vi "M9290A Measure Peak.vi"(7 "Route Names":string[](array[string]), 8 "error in":errorcluster, 10 "Center Frequency (100 MHz)":dbl=1000000000.0, 11 "VISA resource name":refnum<visa-resource-name>="ZVL") -> (0 "error out":errorcluster, 2 "Marker Amplitude (Cal)":dbl, 3 "Marker Amplitude (Raw)":dbl)   [LabVIEW 2015]
uses:
  <instrlib>/Agilent MXA Series/Public/Data/Read Trace (Swept SA).vi
panel:
  out "VISA resource name out":refnum<visa-resource-name>
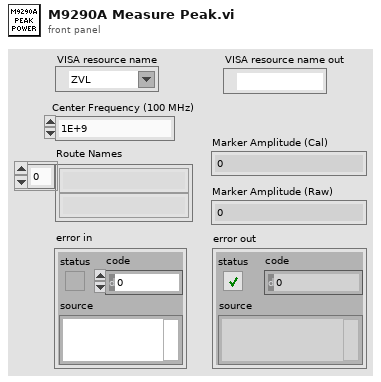
[diagram p1: front panel]
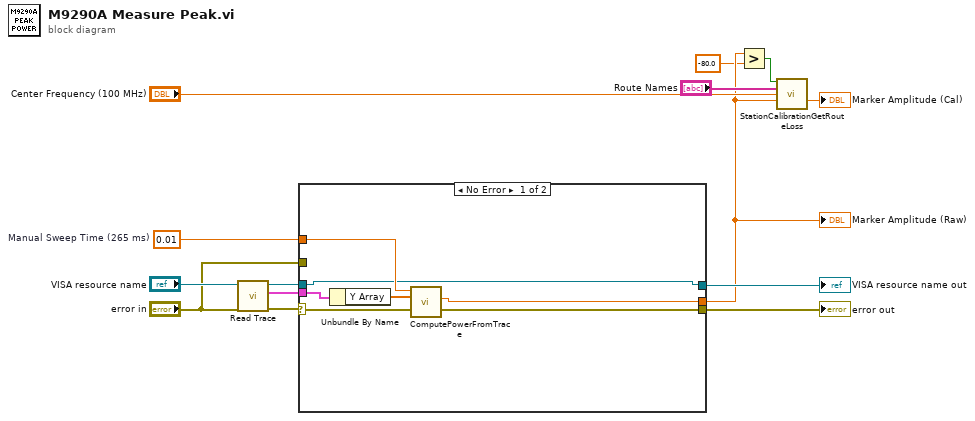
[diagram p0: block diagram]
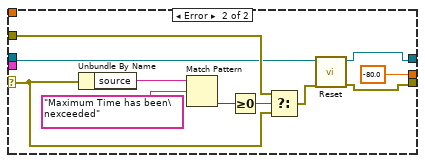
[diagram p2: hidden frame]
diagram:
  w1 = 0.01  # Manual Sweep Time (265 ms)
  n1 = call-poly <instrlib>:"Read Trace.vi"("error in (no error)"="error in", "VISA resource name"="VISA resource name") -> ("error out"=w3:errorcluster, "Trace Waveform"=w2:cluster{"X Array":dbl[], "Y Array":dbl[]}, "VISA resource name out"=w4:refnum<visa-resource-name>)  [unwired: 7 in]
  n2 = case shown="No Error" w3 {
    selector: w3 -> [w16 w25]
    tunnel: [w16 w21] -> w14
    tunnel: [w17 w22] -> w13
    tunnel: [w15 -80.0 ("Marker Amplitude")] -> w7
    tunnel: w4 -> [w17 w23]
    tunnel: "error in" -> [_ w26]
    tunnel: w2 -> [w20 _]
    tunnel: w1 -> [w18 _]
    frame No Error {
      n3 = Unbundle By Name(w20) -> ("Y Array"=w19:dbl[])
      n4 = call "ComputePowerFromTrace.vi"("Trace Array"=w19, "TraceLength"=w18) -> ("Raw Transmit Power"=w15:dbl)  [unwired: 9 in]
    }
    frame Error {
      n5 = Unbundle By Name(w25) -> ("source"=w30:string)
      n6 = Match Pattern(string=w30, regular expression="Maximum Time has been\nexceeded") -> (offset past match=w28:i32)  [unwired: 1 in, 3 out]
      n7 = Greater Or Equal To 0?(x=w28) -> (x >= 0?=w27:bool)
      n8 = Select(t=w26, s=w27, f=w25) -> (s? t:f=w24:errorcluster)
      n9 = call <instrlib>:"Reset.vi"("error in (no error)"=w24, "VISA resource name"=w23) -> ("error out"=w21:errorcluster, "VISA resource name out"=w22:refnum<visa-resource-name>)  [unwired: 8 in]
    }
  }
  "error out" <- w14
  "VISA resource name out" <- w13
  "Marker Amplitude (Raw)" <- w7
  n10 = Greater?(x=w7, y=-80.0) -> (0:w5:bool)
  n11 = call "StationCalibrationGetRouteLoss.vi"("Calibration Enabled"=w5, "Route Names"="Route Names", "Frequency"="Center Frequency (100 MHz)", "Power Level"=w7) -> ("Adjusted Power Level"=→"Marker Amplitude (Cal)":dbl)  [unwired: 8 in, 3 out]
